vi "test_libssh2_channel_get_exit_status.vi"() -> ()   [LabVIEW 2013, in "libssh2_integration_tests.lvlib"]
uses:
  libssh2_integration_tests.lvlib
  <vilib>/addons/_JKI Toolkits/Caraya/classes/Test/Test.lvclass
  libssh2/libssh2.lvlib
  <vilib>/addons/_JKI Toolkits/Caraya/classes/Assert/Assert.lvclass
panel:
  out "error out":errorcluster
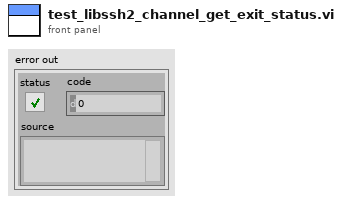
[diagram p1: front panel]
types:
  T1 = typedef "libssh2.lvlib/Session Refnum.ctl" = refnum<k1>
  T2 = typedef "libssh2.lvlib/Channel Refnum.ctl" = refnum<k1>
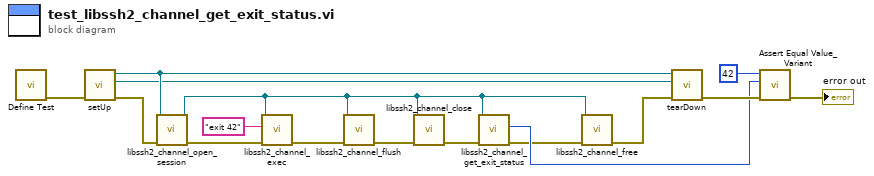
[diagram p0: block diagram]
diagram:
  n1 = call <vilib>:"Define Test.vi"() -> ("error out"=w15:errorcluster)  [unwired: 10 in, 1 out]
  n2 = call "setUp.vi"("error in (no error)"=w15) -> ("error out"=w11:errorcluster, "connection ID"=w12:refnum<k5>, "session"=w13:T1)  [unwired: 8 in]
  n3 = call "libssh2_channel_open_session.vi"("error in (no error)"=w11, "session"=w13) -> ("error out"=w8:errorcluster, "channel"=w1:T2)  [unwired: 8 in]
  n4 = call "libssh2_channel_exec.vi"("error in (no error)"=w8, "command"="exit 42", "channel"=w1) -> ("error out"=w5:errorcluster)  [unwired: 8 in]
  n5 = call "libssh2_channel_flush.vi"("error in (no error)"=w5, "channel"=w1) -> ("error out"=w2:errorcluster)  [unwired: 9 in]
  n6 = call "libssh2_channel_close.vi"("error in (no error)"=w2, "channel"=w1) -> ("error out"=w4:errorcluster)  [unwired: 9 in]
  n7 = call "libssh2_channel_get_exit_status.vi"("error in (no error)"=w4, "channel"=w1) -> ("error out"=w3:errorcluster, "exit status"=w7:i32)  [unwired: 8 in]
  n8 = call "libssh2_channel_free.vi"("error in (no error)"=w3, "channel"=w1) -> ("error out"=w10:errorcluster)  [unwired: 9 in]
  n9 = call "tearDown.vi"("error in (no error)"=w10, "connection ID"=w12, "session"=w13) -> ("error out"=w14:errorcluster)  [unwired: 8 in]
  n10 = call <vilib>:"Assert Equal Value_Variant.vi"("error in (no error)"=w14, "Y"=w7, "X"=42 ("exitsignal")) -> ("error out"=→"error out":errorcluster)  [unwired: 7 in, 1 out]
